vi "JSON_Del_HOOKS.vi"(8 "Error In":errorcluster, 11 "String":string) -> (0 "Error Out":errorcluster, 2 "Array":string[](array[string]), 3 "result string":string)   [LabVIEW 2018]
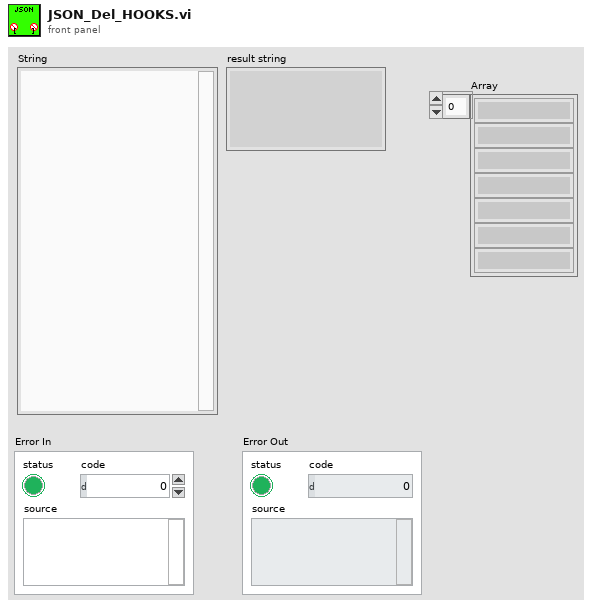
[diagram p1: front panel]
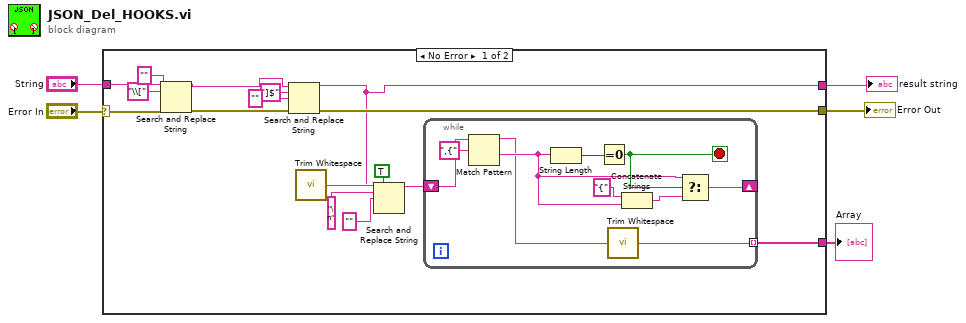
[diagram p0: block diagram]
diagram:
  n1 = case shown="No Error" "Error In" {
    selector: "Error In" -> [w16 w32]
    tunnel: [w7 w33] -> w5
    tunnel: "String" -> [w21 w33]
    tunnel: [w17 w32] -> w2
    tunnel: [w10 _] -> w1
    frame No Error {
      n2 = Search and Replace String(input string=w21, search string="\\[", replace string="" ("replace string (\"\")"), error in=w16) -> (result string=w6:string, error out=w18:errorcluster)  [unwired: 4 in, 2 out]
      n3 = Search and Replace String(input string=w6, search string="]$", replace string="" ("replace string (\"\")"), error in=w18) -> (result string=w7:string, error out=w17:errorcluster)  [unwired: 4 in, 2 out]
      n4 = call <vilib>:"Trim Whitespace.vi"("string"=w7) -> ("trimmed string"=w15:string)  [unwired: 1 in]
      n5 = Search and Replace String(replace all?=TRUE ("replace all? (F)"), input string=w15, search string="\n" ("replace string (\"\")"), replace string="" ("replace string (\"\")")) -> (result string=w11:string)  [unwired: 4 in, 3 out]
      n6 = while {
        shift-right: [w24] -> _
        shift-left: w11 -> [w31]
        tunnel: [w22] -> w10 mode=indexing
        stop <- w28 stop-if-true
        n7 = Match Pattern(string=w31, regular expression=",{") -> (before substring=w23:string, after substring=w25:string)  [unwired: 1 in, 2 out]
        n8 = String Length(string=w25) -> (length=w29:i32)
        n9 = Equal To 0?(x=w29) -> (x = 0?=w28:bool)
        n10 = call <vilib>:"Trim Whitespace.vi"("string"=w23) -> ("trimmed string"=w22:string)  [unwired: 1 in]
        n11 = Concatenate Strings("{" ("regular expression"), w25) -> (w27:string)
        n12 = Select(t=w25, s=w28, f=w27) -> (s? t:f=w24:string)
      }
    }
    frame Error {
    }
  }
  "result string" <- w5
  "Error Out" <- w2
  "Array" <- w1
